vi "Convert to TDM or TDMS.vi"(0 "source file path":path, 1 "DataPlugin name":string, 5 "target file path":path, 7 "target file operation (3:create)":T2=enum."create", 9 "target file format (TDMS)":T1=enum."TDMS", 11 "error in (no error)":errorcluster, 12 "data chunk size (1E+7)":i64=10000000 format="%.0e") -> (3 "DataPlugin name out":string, 4 "source file path out":path, 6 "target file path out":path, 15 "error out":errorcluster)   [LabVIEW 2020]
doc: "Converts the specified file to the .tdm or .tdms file format."
uses:
  <vilib>/Platform/storage/lvStorage.llb/_openFunction.ctl
  <vilib>/Platform/storage/utility/usiTDMTDMS.ctl
  <vilib>/Platform/storage/Storage.llb/Get Property (Storage Refnums).vi
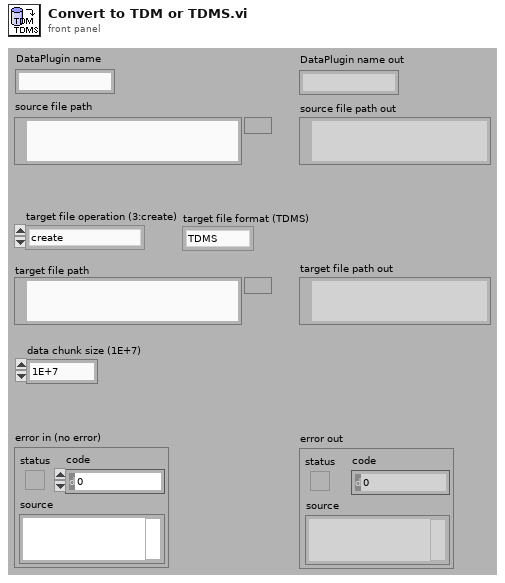
[diagram p1: front panel]
types:
  T1 = typedef "usiTDMTDMS.ctl" = enum16{"TDM", "TDMS"}
  T2 = typedef "_openFunction.ctl" = enum16{"open", "open or create", "create or replace", "create", "open (read only)"}
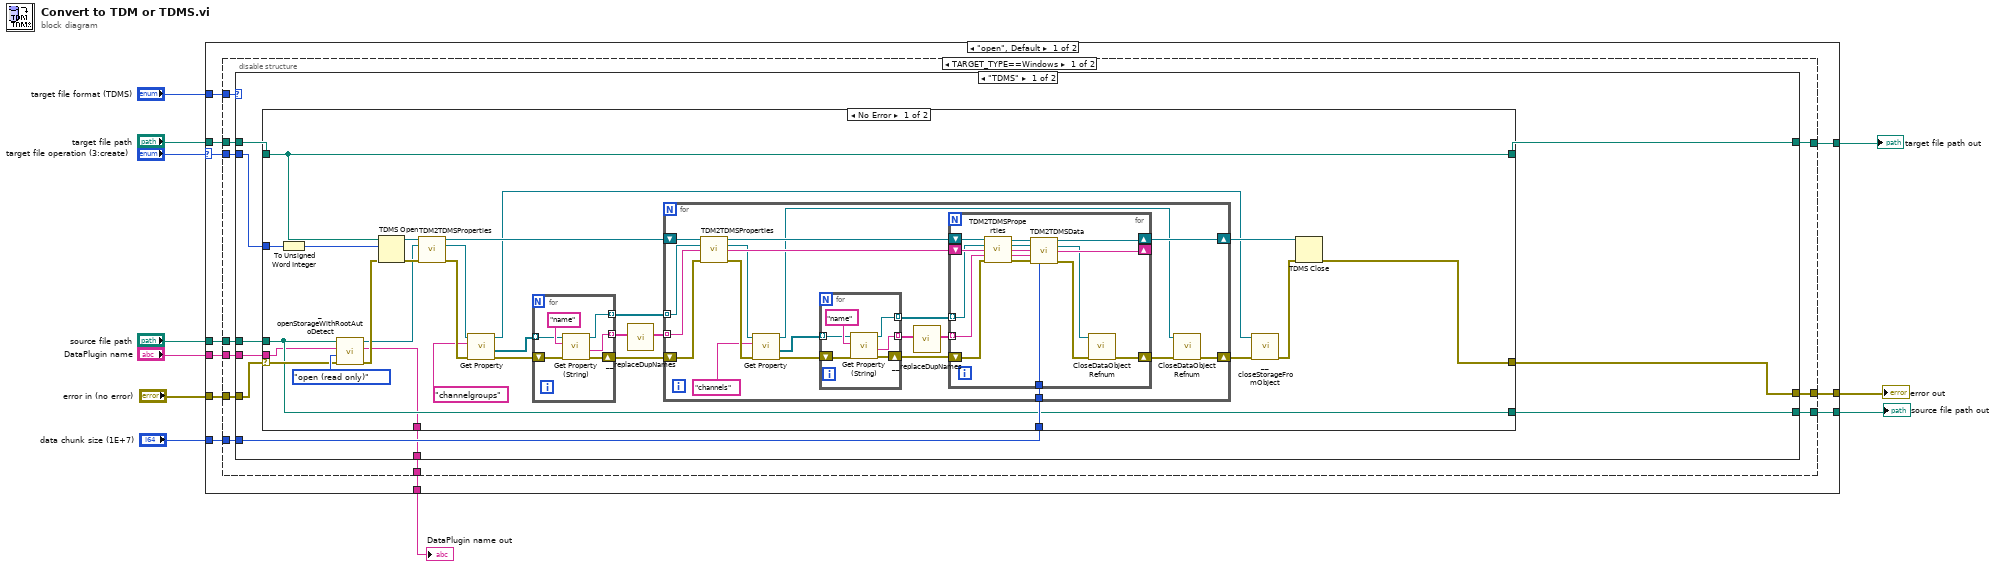
[diagram p0: block diagram]
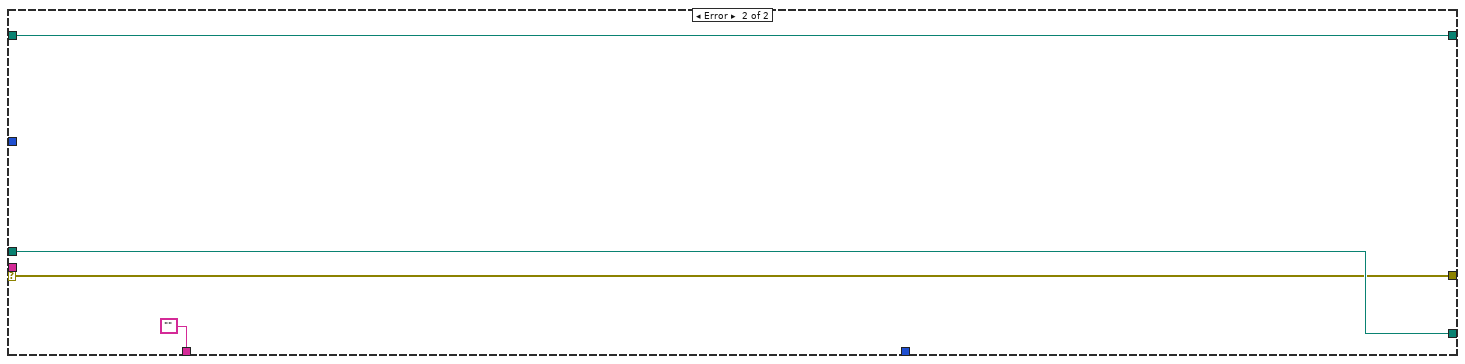
[diagram p2: hidden frame]
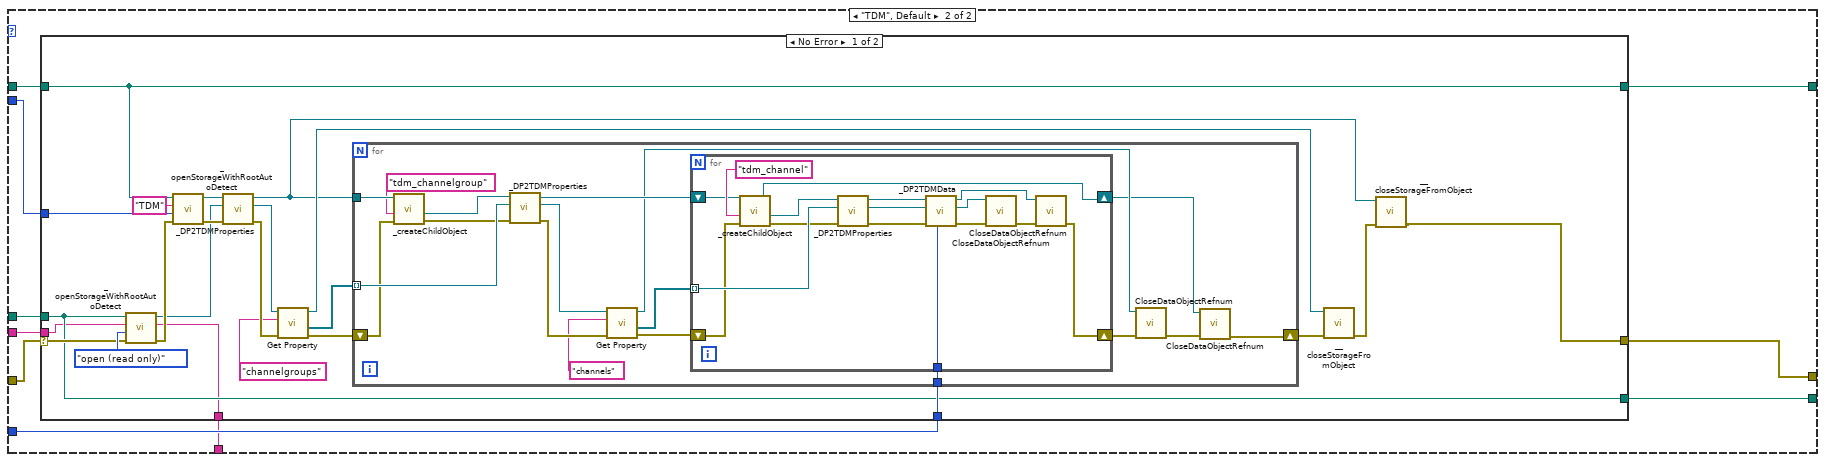
[diagram p3: hidden frame]
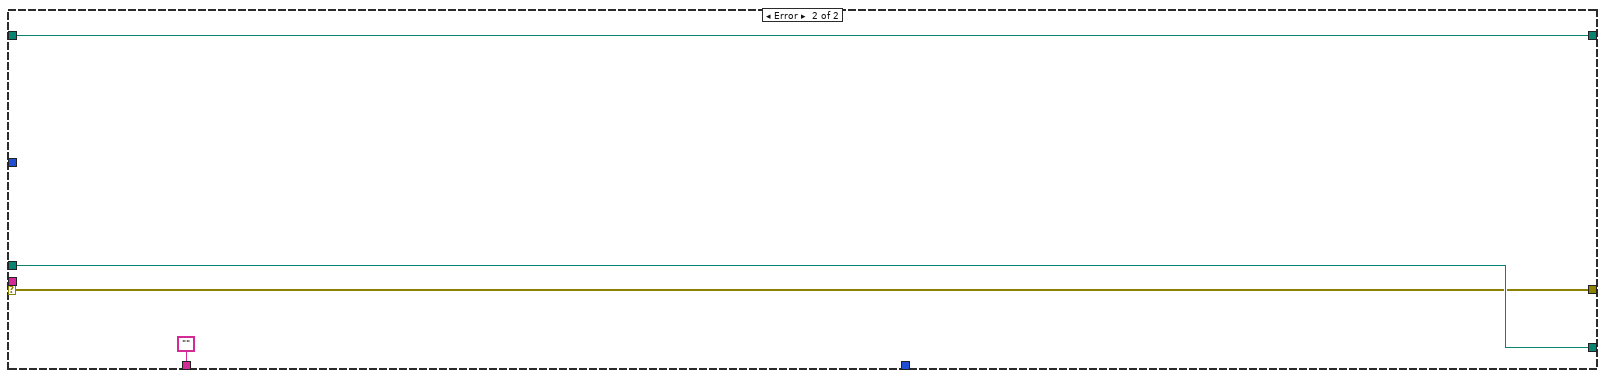
[diagram p4: hidden frame]
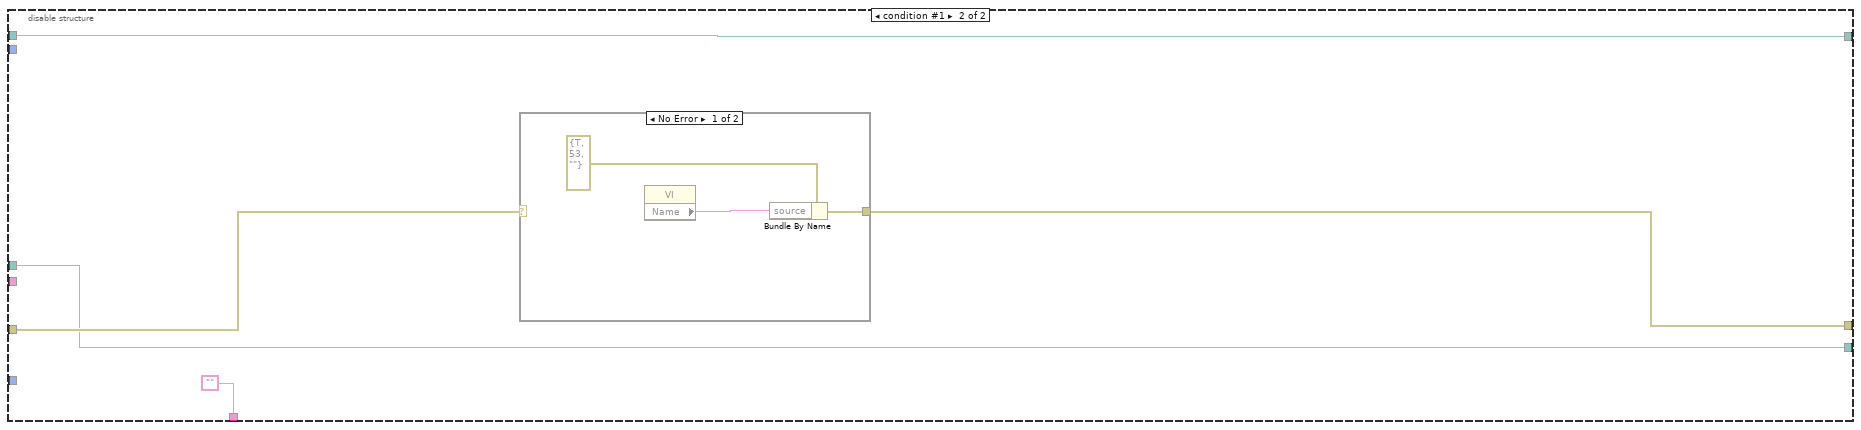
[diagram p5: hidden frame]
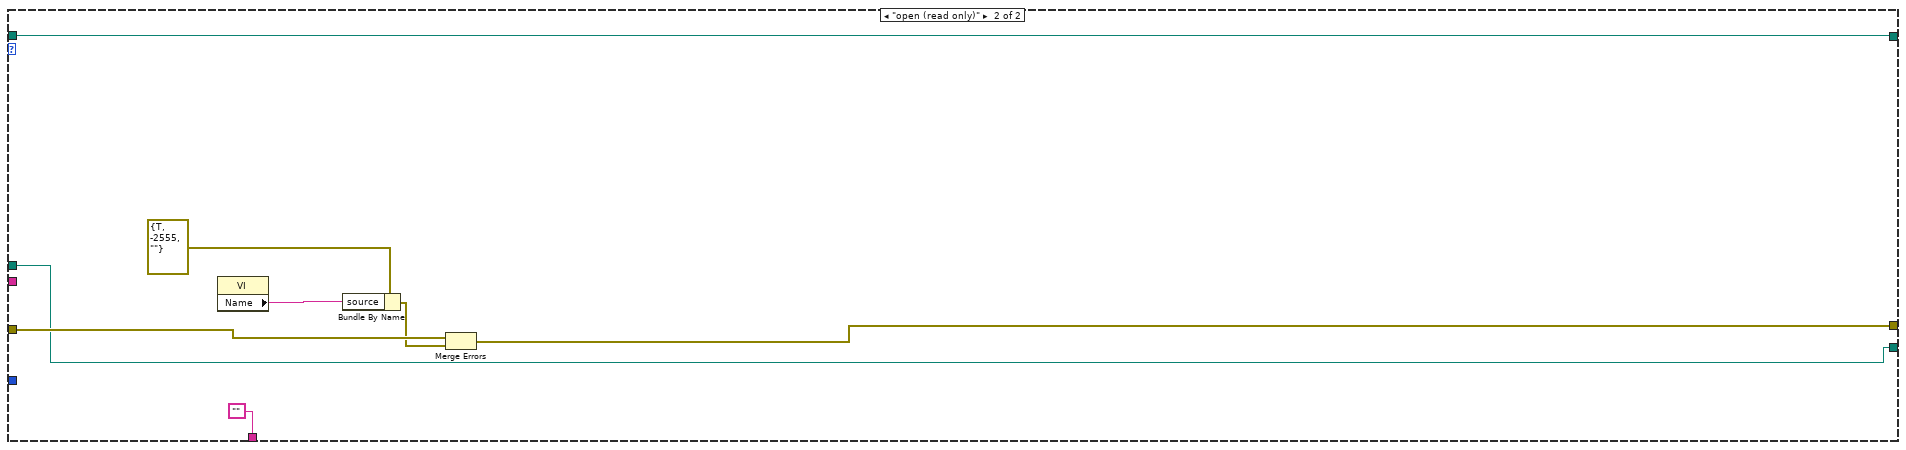
[diagram p7: hidden frame]
diagram:
  n1 = case shown="\"open\", Default" "target file operation (3:create)" {
    selector: "target file operation (3:create)" -> [w19 _]
    tunnel: "target file format (TDMS)" -> [w22 _]
    tunnel: "error in (no error)" -> [w20 w211]
    tunnel: [w15 w210] -> w4
    tunnel: "target file path" -> [w21 w206]
    tunnel: "DataPlugin name" -> [w18 _]
    tunnel: "source file path" -> [w17 w205]
    tunnel: "data chunk size (1E+7)" -> [w16 _]
    tunnel: [w14 w206] -> w3
    tunnel: [w13 w205] -> w2
    tunnel: [w12 "" ("Storage Format out")] -> w1
    frame "open", Default {
      n2 = disable-structure shown="TARGET_TYPE==Windows" {
        disable-tunnel: w22 -> [w33 _]
        disable-tunnel: w21 -> [w32 w197]
        disable-tunnel: w20 -> [w31 w199]
        disable-tunnel: w19 -> [w30 _]
        disable-tunnel: w18 -> [w29 _]
        disable-tunnel: w17 -> [w28 w196]
        disable-tunnel: w16 -> [w27 _]
        disable-tunnel: [w26 w198] -> w15
        disable-tunnel: [w24 w197] -> w14
        disable-tunnel: [w25 w196] -> w13
        disable-tunnel: [w23 "" ("Storage Format out")] -> w12
        frame condition #0 (active) {
          n3 = case shown="\"TDMS\"" w33 {
            tunnel: w32 -> [w42 w132]
            tunnel: w31 -> [w43 w133]
            tunnel: w30 -> [w41 w131]
            tunnel: w29 -> [w39 w129]
            tunnel: w28 -> [w40 w130]
            tunnel: w27 -> [w38 w128]
            tunnel: [w37 w127] -> w26
            tunnel: [w36 w126] -> w25
            tunnel: [w35 w125] -> w24
            tunnel: [w34 w124] -> w23
            frame "TDMS" {
              n4 = case shown="No Error" w43 {
                selector: w43 -> [w63 w121]
                tunnel: w41 -> [w69 _]
                tunnel: [w44 w121] -> w37
                tunnel: w40 -> [w60 w122]
                tunnel: w42 -> [w59 w123]
                tunnel: [w59 w123] -> w35
                tunnel: [w60 w122] -> w36
                tunnel: w38 -> [w61 _]
                tunnel: w39 -> [w46 _]
                tunnel: [w45 "" ("Storage Format out")] -> w34
                frame No Error {
                  n5 = To Unsigned Word Integer(number=w69) -> (unsigned 16bit integer=w47:u16)
                  n6 = call <vilib>:"_openStorageWithRootAutoDetect.vi"("error in (no error)"=w63, "Overwrite Options"=_openFunction."open (read only)", "Storage Format"=w46, "Storage Location"=w60) -> ("error out"=w62:errorcluster, "Storage Format out"=w45:string, "Data Object"=w54:refnum<k20>)  [unwired: 5 in]
                  n7 = TDMS Open(8:w62, 10:w47, 11:w59) -> (0:w71:errorcluster, 3:w68:refnum<k34>)  [unwired: 4 in]
                  n8 = call <vilib>:"TDM2TDMSProperties.vi"("tdms file in"=w68, "Data Object in"=w54, "error in (no error)"=w71) -> ("tdms file out"=w70:refnum<k34>, "Data Object out"=w58:refnum<k20>, "error out"=w57:errorcluster)  [unwired: 8 in, 2 out]
                  n9 = call-poly <vilib>:"Get Property.vi"("error in (no error)"=w57, "Property name"="channelgroups", "storage refnum"=w58) -> ("error out"=w53:errorcluster, "Value"=w52:refnum<k20>[], "storage refnum out"=w56:refnum<k20>)  [unwired: 6 in]
                  n10 = for {
                    shift-right: [w76] -> w50
                    shift-left: w53 -> [w75]
                    tunnel: w52 -> [w74] mode=indexing
                    tunnel: [w73] -> w51 mode=indexing
                    tunnel: [w72] -> w49 mode=indexing
                    n11 = call <vilib>:"Get Property (String).vi"("error in (no error)"=w75, "Property name"="name", "storage refnum"=w74) -> ("error out"=w76:errorcluster, "Value"=w72:string, "storage refnum out"=w73:refnum<k20>)  [unwired: 6 in]
                  }
                  n12 = call <vilib>:"__replaceDupNames.vi"("input names"=w49) -> ("output names"=w48:string[])  [unwired: 10 in]
                  n13 = for {
                    shift-right: [w95] -> w64
                    shift-left: w70 -> [w97]
                    shift-right: [w79] -> w66
                    shift-left: w50 -> [w82]
                    tunnel: w61 -> [w93]
                    tunnel: w51 -> [w81] mode=indexing
                    tunnel: w48 -> [w83] mode=indexing
                    n14 = call <vilib>:"TDM2TDMSProperties.vi"("tdms file in"=w97, "Data Object in"=w81, "group name"=w83, "error in (no error)"=w82) -> ("tdms file out"=w96:refnum<k34>, "Data Object out"=w90:refnum<k20>, "group name out"=w94:string, "error out"=w92:errorcluster)  [unwired: 7 in, 1 out]
                    n15 = call-poly <vilib>:"Get Property.vi"("error in (no error)"=w92, "Property name"="channels", "storage refnum"=w90) -> ("error out"=w89:errorcluster, "Value"=w88:refnum<k20>[], "storage refnum out"=w78:refnum<k20>)  [unwired: 6 in]
                    n16 = for {
                      shift-right: [w101] -> w87
                      shift-left: w89 -> [w102]
                      tunnel: w88 -> [w100] mode=indexing
                      tunnel: [w99] -> w86 mode=indexing
                      tunnel: [w98] -> w84 mode=indexing
                      n17 = call <vilib>:"Get Property (String).vi"("error in (no error)"=w102, "Property name"="name", "storage refnum"=w100) -> ("error out"=w101:errorcluster, "Value"=w99:string, "storage refnum out"=w98:refnum<k20>)  [unwired: 6 in]
                    }
                    n18 = call <vilib>:"__replaceDupNames.vi"("input names"=w86) -> ("output names"=w85:string[])  [unwired: 10 in]
                    n19 = for {
                      shift-right: [w115] -> w95
                      shift-left: w96 -> [w118]
                      shift-right: [w106] -> w80
                      shift-left: w87 -> [w108]
                      tunnel: w93 -> [w111]
                      shift-right: [w110] -> _
                      shift-left: w94 -> [w119]
                      tunnel: w85 -> [w107] mode=indexing
                      tunnel: w84 -> [w109] mode=indexing
                      n20 = call <vilib>:"TDM2TDMSProperties.vi"("tdms file in"=w118, "Data Object in"=w109, "group name"=w119, "channel name"=w107, "error in (no error)"=w108) -> ("tdms file out"=w117:refnum<k34>, "Data Object out"=w116:refnum<k20>, "group name out"=w113:string, "channel name out"=w112:string, "error out"=w114:errorcluster)  [unwired: 6 in]
                      n21 = call <vilib>:"TDM2TDMSData.vi"("tdms file in"=w117, "storage refnum in"=w116, "group name"=w113, "channel name"=w112, "error in (no error)"=w114, "chunk size"=w111) -> ("tdms file out"=w115:refnum<k34>, "storage refnum out"=w104:refnum<k20>, "group name out"=w110:string, "error out"=w105:errorcluster)  [unwired: 5 in, 1 out]
                      n22 = call <vilib>:"CloseDataObjectRefnum.vi"("error in (no error)"=w105, "storage refnum"=w104) -> ("error out"=w106:errorcluster)  [unwired: 9 in]
                    }
                    n23 = call <vilib>:"CloseDataObjectRefnum.vi"("error in (no error)"=w80, "storage refnum"=w78) -> ("error out"=w79:errorcluster)  [unwired: 9 in]
                  }
                  n24 = call <vilib>:"__closeStorageFromObject.vi"("error in (no error)"=w66, "storage refnum"=w56) -> ("error out"=w65:errorcluster)  [unwired: 5 in]
                  n25 = TDMS Close(8:w65, 11:w64) -> (0:w44:errorcluster)  [unwired: 1 out]
                }
                frame Error {
                }
              }
            }
            frame "TDM", Default {
              n26 = case shown="No Error" w133 {
                selector: w133 -> [w154 w192]
                tunnel: w131 -> [w148 _]
                tunnel: [w134 w192] -> w127
                tunnel: w130 -> [w152 w193]
                tunnel: w132 -> [w149 w194]
                tunnel: [w149 w194] -> w125
                tunnel: [w152 w193] -> w126
                tunnel: w128 -> [w153 _]
                tunnel: w129 -> [w150 _]
                tunnel: [w137 "" ("Storage Format out")] -> w124
                frame No Error {
                  n27 = call <vilib>:"_openStorageWithRootAutoDetect.vi"("error in (no error)"=w154, "Overwrite Options"=_openFunction."open (read only)", "Storage Format"=w150, "Storage Location"=w152) -> ("error out"=w146:errorcluster, "Storage Format out"=w137:string, "Data Object"=w143:refnum<k20>)  [unwired: 5 in]
                  n28 = call <vilib>:"_openStorageWithRootAutoDetect.vi"("error in (no error)"=w146, "Overwrite Options"=w148, "Storage Format"="TDM", "Storage Location"=w149) -> ("error out"=w145:errorcluster, "Data Object"=w144:refnum<k20>)  [unwired: 5 in, 1 out]
                  n29 = call <vilib>:"_DP2TDMProperties.vi"("error in (no error)"=w145, "DataPlugin Object in"=w143, "TDM Object in"=w144) -> ("error out"=w142:errorcluster, "DataPlugin object out"=w141:refnum<k20>, "TDM Object out"=w135:refnum<k20>)  [unwired: 6 in]
                  n30 = call-poly <vilib>:"Get Property.vi"("error in (no error)"=w142, "Property name"="channelgroups", "storage refnum"=w141) -> ("error out"=w136:errorcluster, "Value"=w139:refnum<k20>[], "storage refnum out"=w151:refnum<k20>)  [unwired: 6 in]
                  n31 = for {
                    shift-right: [w158] -> w155
                    shift-left: w136 -> [w167]
                    tunnel: w153 -> [w174]
                    tunnel: w139 -> [w173] mode=indexing
                    tunnel: w135 -> [w168]
                    n32 = call <vilib>:"_createChildObject.vi"("error in (no error)"=w167, "Object type"="tdm_channelgroup", "storage refnum"=w168) -> ("error out"=w165:errorcluster, "new storage refnum"=w164:refnum<k20>)  [unwired: 2 in, 1 out]
                    n33 = call <vilib>:"_DP2TDMProperties.vi"("error in (no error)"=w165, "DataPlugin Object in"=w173, "TDM Object in"=w164) -> ("error out"=w172:errorcluster, "DataPlugin object out"=w171:refnum<k20>, "TDM Object out"=w162:refnum<k20>)  [unwired: 6 in]
                    n34 = call-poly <vilib>:"Get Property.vi"("error in (no error)"=w172, "Property name"="channels", "storage refnum"=w171) -> ("error out"=w163:errorcluster, "Value"=w169:refnum<k20>[], "storage refnum out"=w161:refnum<k20>)  [unwired: 6 in]
                    n35 = for {
                      shift-right: [w176] -> w160
                      shift-left: w163 -> [w185]
                      tunnel: w174 -> [w189]
                      tunnel: w169 -> [w190] mode=indexing
                      shift-right: [w175] -> w157
                      shift-left: w162 -> [w181]
                      n36 = call <vilib>:"_createChildObject.vi"("error in (no error)"=w185, "Object type"="tdm_channel", "storage refnum"=w181) -> ("error out"=w183:errorcluster, "new storage refnum"=w182:refnum<k20>, "dup storage refnum"=w175:refnum<k20>)  [unwired: 2 in]
                      n37 = call <vilib>:"_DP2TDMProperties.vi"("error in (no error)"=w183, "DataPlugin Object in"=w190, "TDM Object in"=w182) -> ("error out"=w188:errorcluster, "DataPlugin object out"=w186:refnum<k20>, "TDM Object out"=w187:refnum<k20>)  [unwired: 6 in]
                      n38 = call <vilib>:"_DP2TDMData.vi"("chunk size"=w189, "error in (no error)"=w188, "DataPlugin Object in"=w186, "TDM Object in"=w187) -> ("error out"=w179:errorcluster, "DataPlugin object out"=w180:refnum<k20>, "TDM Object out"=w177:refnum<k20>)  [unwired: 5 in]
                      n39 = call <vilib>:"CloseDataObjectRefnum.vi"("error in (no error)"=w179, "storage refnum"=w180) -> ("error out"=w178:errorcluster)  [unwired: 9 in]
                      n40 = call <vilib>:"CloseDataObjectRefnum.vi"("error in (no error)"=w178, "storage refnum"=w177) -> ("error out"=w176:errorcluster)  [unwired: 9 in]
                    }
                    n41 = call <vilib>:"CloseDataObjectRefnum.vi"("error in (no error)"=w160, "storage refnum"=w161) -> ("error out"=w159:errorcluster)  [unwired: 9 in]
                    n42 = call <vilib>:"CloseDataObjectRefnum.vi"("error in (no error)"=w159, "storage refnum"=w157) -> ("error out"=w158:errorcluster)  [unwired: 9 in]
                  }
                  n43 = call <vilib>:"__closeStorageFromObject.vi"("error in (no error)"=w155, "storage refnum"=w151) -> ("error out"=w140:errorcluster)  [unwired: 5 in]
                  n44 = call <vilib>:"__closeStorageFromObject.vi"("error in (no error)"=w140, "storage refnum"=w135) -> ("error out"=w134:errorcluster)  [unwired: 5 in]
                }
                frame Error {
                }
              }
            }
          }
        }
        frame condition #1 {
          n45 = case shown="No Error" w199 {
            selector: w199 -> [_ w203]
            tunnel: [w201 w203] -> w198
            frame No Error {
              n46 = property class="VI"() -> ("Name"=w200:string)  [unwired: 2 in, 2 out]
              n47 = Bundle By Name(cluster=errorcluster {"status"=TRUE, "code"=53, "source"=""} ("error IO"), "source"=w200) -> (w201:errorcluster)
            }
            frame Error {
            }
          }
        }
      }
    }
    frame "open (read only)" {
      n48 = property class="VI"() -> ("Name"=w209:string)  [unwired: 2 in, 2 out]
      n49 = Bundle By Name(cluster=errorcluster {"status"=TRUE, "code"=-2555, "source"=""} ("error in 2 (no error)"), "source"=w209) -> (w207:errorcluster)
      n50 = Merge Errors(w211, w207) -> (w210:errorcluster)
    }
  }
  "error out" <- w4
  "source file path out" <- w2
  "target file path out" <- w3
  "DataPlugin name out" <- w1
